vi "read digital HP.vi"(8 "error in (no error)":errorcluster, 11 "ID":i32) -> (0 "error out":errorcluster, 3 "Digital Signal":T1={"DAQ Board Name"="DAQ_Simu1", "Port Digitales"=[], "rate"=1000.0, "Tiempo"=100})   [LabVIEW 2020, in "Settings.lvlib"]
uses:
  Settings.lvlib
  Digital typeSignal--cluster.ctl
  <vilib>/drjdpowell/SQLite Library/SQL Connection/Open (path).vi
  <vilib>/drjdpowell/SQLite Library/SQL Connection/Open (string).vi
  <vilib>/AdvancedString/Path To Command Line String.vi
  <vilib>/drjdpowell/SQLite Library/SQL Connection/Execute SQL (1D UTF-8).vi
  <vilib>/drjdpowell/SQLite Library/SQL Connection/Connection.lvclass
  <vilib>/drjdpowell/SQLite Library/SQLite.lvlib
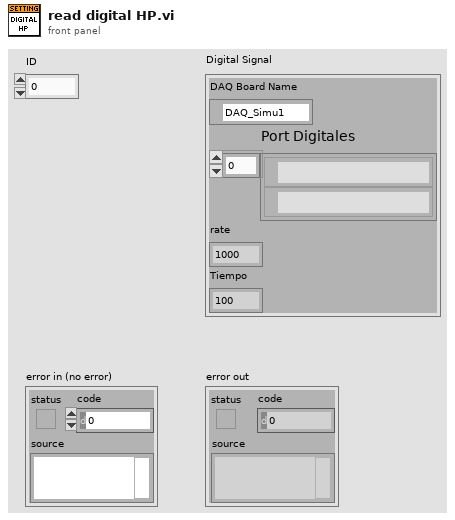
[diagram p1: front panel]
types:
  T1 = typedef "Digital typeSignal--cluster.ctl" = cluster{"DAQ Board Name":tag, "Port Digitales":tag[], "rate":dbl, "Tiempo":i32}
  T2 = cluster{"Result Set (UTF-8)[0]":string, "Result Set (UTF-8)[1]":string, "Result Set (UTF-8)[2]":string, "Result Set (UTF-8)[3]":string, "Result Set (UTF-8)[4]":string, "Result Set (UTF-8)[5]":string, "Result Set (UTF-8)[6]":string, "Result Set (UTF-8)[7]":string, "Result Set (UTF-8)[8]":string}
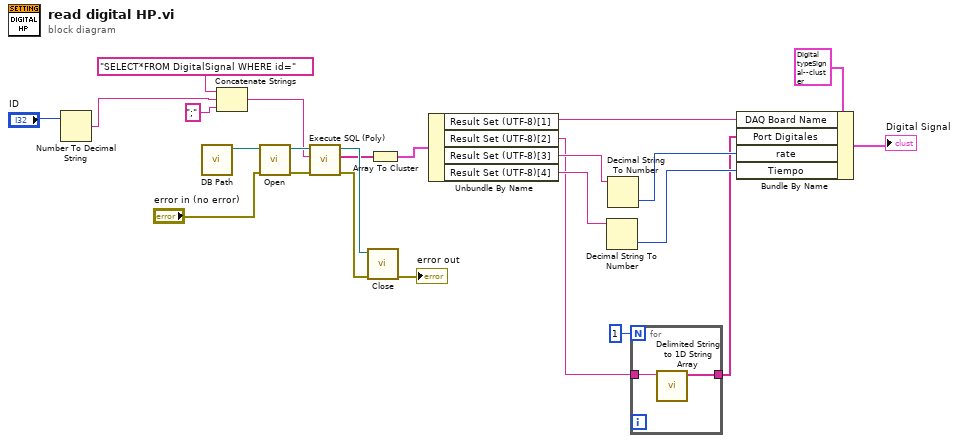
[diagram p0: block diagram]
diagram:
  n1 = Number To Decimal String(number="ID") -> (decimal integer string=w11:string)  [unwired: 1 in]
  n2 = call "DB Path.vi"() -> ("DB path"=w16:path)  [unwired: 11 in]
  n3 = Concatenate Strings("SELECT*FROM DigitalSignal WHERE id=" ("SQL"), w11, ";" ("string")) -> (w13:string)
  n4 = call-poly <vilib>:"Open.vi"("error in (no error)"="error in (no error)", "db file"=w16) -> ("error out"=w24:errorcluster, "SQLite Connection"=w23:refnum<class "Connection.lvclass">)  [unwired: 8 in]
  n5 = call-poly <vilib>:"Execute SQL (Poly).vi"("error in (no error)"=w24, "SQL"=w13, "SQLite Connection in"=w23) -> ("error out"=w21:errorcluster, "Result Set (UTF-8)"=w17:string[], "SQLite Connection"=w22:refnum<class "Connection.lvclass">)  [unwired: 5 in, 1 out]
  n6 = call-dynamic "Close.vi"("error in (no error)"=w21, "SQLite Connection in"=w22) -> ("error out"=→"error out":errorcluster)  [unwired: 9 in]
  n7 = Array To Cluster(array=w17) -> (cluster=w18:T2)
  n8 = Unbundle By Name(w18) -> ("Result Set (UTF-8)[1]"=w7:string, "Result Set (UTF-8)[2]"=w2:string, "Result Set (UTF-8)[3]"=w6:string, "Result Set (UTF-8)[4]"=w5:string)
  n9 = Decimal String To Number(string=w5) -> (number=w9:i32)  [unwired: 2 in, 1 out]
  n10 = Decimal String To Number(string=w6) -> (number=w10:i32)  [unwired: 2 in, 1 out]
  n11 = for {
    N: 1 -> [_]
    tunnel: [w26] -> w1
    tunnel: w2 -> [w25]
    n12 = call <vilib>:"Delimited String to 1D String Array.vi"("delimited string"=w25) -> ("string array"=w26:string[])  [unwired: 10 in]
  }
  n13 = Bundle By Name(cluster=T1 {"DAQ Board Name"="DAQ_Simul2", "Port Digitales"=["DAQ_Simul2/port0", "\t", "\t", "\t", "\t", "\t", "\t", "\t"], "rate"=100.0, "Tiempo"=2} ("Digital Signal"), "DAQ Board Name"=w7, "Port Digitales"=w1, "rate"=w10, "Tiempo"=w9) -> (→"Digital Signal":T1)
